vi "LiXiang's SRAM TESTING.vi"(8 "error in (no error)":errorcluster, 11 "DATA PATTERN":u8) -> (0 "错误输出":errorcluster, 3 "SEU number":u32)   [LabVIEW 2015]
doc: "演示连接TCP服务器、读取发送的数据并在图表上显示数据的方法。VI设计为TCP连接断开时停止。"
panel:
  out "布尔":bool
  out "SEU？":bool
  out "数组 2":i32[][](array[numeric])
  in  "行":u32
  out "数据输出":string
  in  "停止":bool
  # "地址"
  # "数据"
  # "0: 00\n1: 10\n2: 11"
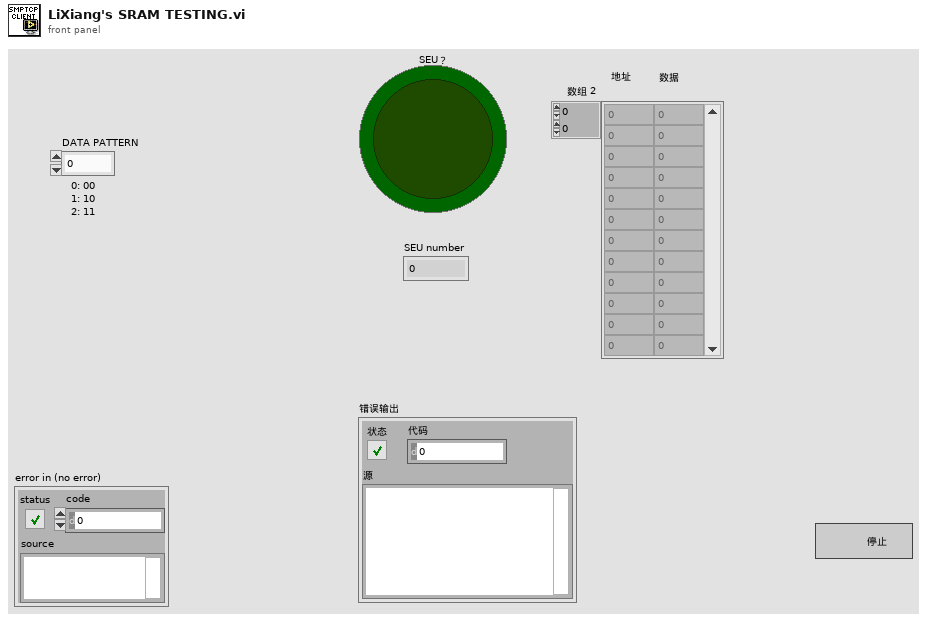
[diagram p1: front panel]
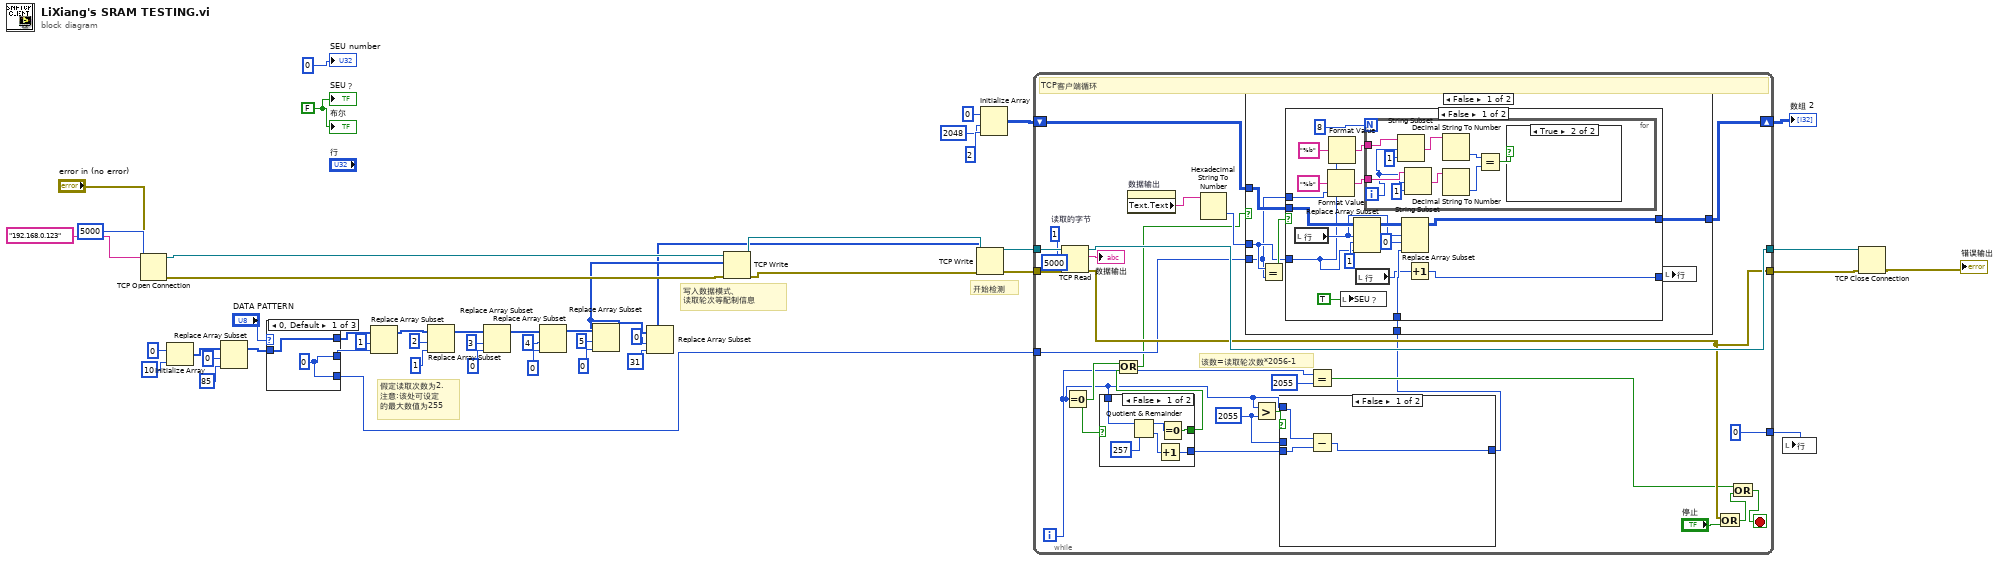
[diagram p0: block diagram]
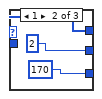
[diagram p2: hidden frame]
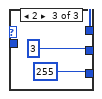
[diagram p3: hidden frame]
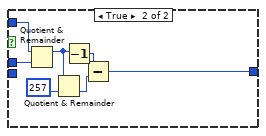
[diagram p4: hidden frame]
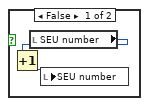
[diagram p5: hidden frame]
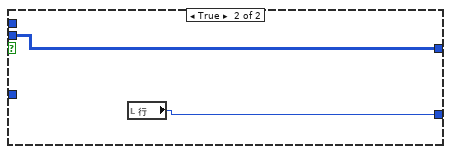
[diagram p6: hidden frame]
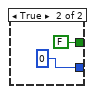
[diagram p8: hidden frame]
diagram:
  w7 = FALSE ("布尔")
  # "开始检测"
  # "写入数据模式、\n读取轮次等配制信息"
  # "假定读取次数为2.\n注意:该处可设定\n的最大数值为255"
  n1 = TCP Open Connection(address="192.168.0.123" ("地址"), remote port or service name=u16 5000 ("端口"), error in (no error)="error in (no error)") -> (connection ID=w25:refnum<k5>, error out=w24:errorcluster)  [unwired: 2 in]
  n2 = Initialize Array(u8 0 ("元素"), 10 ("维数大小")) -> (w43:u8[])
  n3 = Replace Array Subset(array=w43, new element=u8 85 ("新元素/子数组"), index=0 ("索引")) -> (w40:u8[])
  n4 = case shown="0, Default" "DATA PATTERN" {
    tunnel: w40 -> [w49 w52 w55]
    tunnel: [w49 w52 w55] -> w27
    tunnel: [w48 u8 2 ("新元素/子数组") u8 3 ("新元素/子数组")] -> w8
    tunnel: [w48 u32 170 ("新元素/子数组") u32 255 ("新元素/子数组")] -> w10
    frame 0, Default {
      w48 = u8 0 ("新元素/子数组")
    }
    frame 1 {
    }
    frame 2 {
    }
  }
  n5 = Replace Array Subset(array=w27, new element=w8, index=1 ("索引")) -> (w26:u8[])
  n6 = Replace Array Subset(array=w26, new element=u8 1 ("新元素/子数组"), index=2 ("索引")) -> (w36:u8[])
  n7 = Replace Array Subset(array=w36, new element=u8 0 ("新元素/子数组"), index=3 ("索引")) -> (w33:u8[])
  n8 = Replace Array Subset(array=w33, new element=u8 0 ("新元素/子数组"), index=4 ("索引")) -> (w30:u8[])
  n9 = Replace Array Subset(array=w30, new element=u8 0 ("新元素/子数组"), index=5 ("索引")) -> (w18:u8[])
  n10 = Replace Array Subset(array=w18, new element=u8 31 ("新元素/子数组"), index=0 ("索引")) -> (w17:u8[])
  n11 = TCP Write(connection ID=w25, data in=w18, error in (no error)=w24) -> (connection ID out=w23:refnum<k5>, error out=w5:errorcluster)  [unwired: 1 in, 1 out]
  n12 = TCP Write(connection ID=w23, data in=w17, error in (no error)=w5) -> (connection ID out=w21:refnum<k5>, error out=w22:errorcluster)  [unwired: 1 in, 1 out]
  n13 = Initialize Array(0 ("元素"), 2048 ("维数大小"), 2 ("维数大小")) -> (w12:i32[][])
  n14 = while {
    tunnel: w22 -> [w80]
    tunnel: w21 -> [w81]
    tunnel: [w77] -> w1
    tunnel: [w76] -> w3
    tunnel: w10 -> [w69]
    shift-right: [w62] -> w6
    shift-left: w12 -> [w65]
    tunnel: [u32 0 ("行")] -> w11
    i -> [w60]
    stop <- w73 stop-if-true
    w63 = 2055 ("y")
    w79 = 1  # 读取的字节
    # "该数=读取轮次数*2056-1"
    # "TCP客户端循环"
    n15 = TCP Read(connection ID=w81, bytes to read=w79, error in (no error)=w80, 9:5000 ("超时毫秒(25000)")) -> (connection ID out=w77:refnum<k5>, data out=→"数据输出":string, error out=w76:errorcluster)  [unwired: 1 in]
    n16 = Equal To 0?(x=w60) -> (x = 0?=w68:bool)
    n17 = case shown="False" w68 {
      tunnel: w60 -> [w131 _]
      tunnel: [w134 FALSE] -> w67
      tunnel: [w132 0] -> w58
      frame False {
        n18 = Quotient & Remainder(x=w131, y=257) -> (x-y*floor(x/y)=w135:i32, floor(x/y)=w133:i32)
        n19 = Increment(x=w133) -> (x+1=w132:i32)
        n20 = Equal To 0?(x=w135) -> (x = 0?=w134:bool)
      }
      frame True {
      }
    }
    n21 = Or(x=w68, y=w67) -> (x .or. y?=w66:bool)
    n22 = property on="数据输出" class="Str"() -> ("Text.Text"=w57:string)  [unwired: 2 in, 2 out]
    n23 = Hexadecimal String To Number(string=w57) -> (number=w70:u32)  [unwired: 2 in, 1 out]
    n24 = Greater?(x=w60, y=w63) -> (0:w64:bool)
    n25 = case shown="False" w64 {
      tunnel: w60 -> [w82 w91]
      tunnel: w63 -> [_ w90]
      tunnel: [w83 w86] -> w59
      tunnel: w58 -> [w84 _]
      frame False {
        n26 = Subtract(x=w82, y=w84) -> (x-y=w83:i32)
      }
      frame True {
        n27 = Quotient & Remainder(x=w91, y=w90) -> (x-y*floor(x/y)=w89:i32)  [unwired: 1 out]
        n28 = Quotient & Remainder(x=w89, y=257) -> (floor(x/y)=w87:i32)  [unwired: 1 out]
        n29 = Decrement(x=w89) -> (x-1=w85:i32)
        n30 = Subtract(x=w85, y=w87) -> (x-y=w86:i32)
      }
    }
    n31 = case shown="False" w66 {
      tunnel: w70 -> [w95 _]
      tunnel: w69 -> [w92 _]
      tunnel: w65 -> [w97 w130]
      tunnel: w59 -> [w96 _]
      tunnel: [w94 w130] -> w62
      frame False {
        n32 = Equal?(x=w95, y=w92) -> (x = y?=w98:bool)
        n33 = case shown="False" w98 {
          tunnel: w97 -> [w115 w129]
          tunnel: w96 -> [w110 _]
          tunnel: w95 -> [w103 _]
          tunnel: [w109 w129] -> w94
          tunnel: [w107 w128] -> w93
          tunnel: w92 -> [w100 _]
          frame False {
            n34 = local read "行"() -> (w112:u32)
            n35 = Format Value(format string="%b" ("格式字符串"), value (0)=w100) -> (output string=w99:string)  [unwired: 1 in]
            n36 = Format Value(format string="%b" ("格式字符串"), value (0)=w103) -> (output string=w102:string)  [unwired: 1 in]
            n37 = local write "SEU？"(TRUE ("SEU？")) -> ()
            n38 = Replace Array Subset(array=w115, new element=w103, index (row)=w112, index (col)=1 ("禁用的索引 (列)")) -> (w113:i32[][])
            n39 = local read "行"() -> (w108:u32)
            n40 = for {
              N: 8 -> [_]
              tunnel: w102 -> [w125]
              tunnel: w99 -> [w121]
              i -> [w120]
              n41 = String Subset(string=w125, offset (0)=w120, length (rest)=1 ("长度（剩余）")) -> (substring=w123:string)
              n42 = String Subset(string=w121, offset (0)=w120, length (rest)=1 ("长度（剩余）")) -> (substring=w119:string)
              n43 = Decimal String To Number(string=w123) -> (number=w118:i32)  [unwired: 2 in, 1 out]
              n44 = Decimal String To Number(string=w119) -> (number=w117:i32)  [unwired: 2 in, 1 out]
              n45 = Equal?(x=w118, y=w117) -> (x = y?=w116:bool)
              n46 = case shown="True" w116 {
                frame False {
                  n47 = local read "SEU number"() -> (w127:u32)
                  n48 = Increment(x=w127) -> (x+1=w126:u32)
                  n49 = local write "SEU number"(w126) -> ()
                }
                frame True {
                }
              }
            }
            n50 = Replace Array Subset(array=w113, new element=w110, index (row)=w112, index (col)=0 ("禁用的索引 (列)")) -> (w109:i32[][])
            n51 = Increment(x=w108) -> (x+1=w107:u32)
          }
          frame True {
            n52 = local read "行"() -> (w128:u32)
          }
        }
        n53 = local write "行"(w93) -> ()
      }
      frame True {
      }
    }
    n54 = Equal?(x=w60, y=2055) -> (x = y?=w75:bool)
    n55 = Or(x=w76, y="停止") -> (x .or. y?=w74:bool)
    n56 = Or(x=w75, y=w74) -> (x .or. y?=w73:bool)
  }
  "数组 2" <- w6
  n57 = local write "行"(w11) -> ()
  n58 = TCP Close Connection(connection ID=w1, error in (no error)=w3) -> (error out=→"错误输出":errorcluster)  [unwired: 1 in, 1 out]
  "SEU？" <- w7
  "SEU number" <- u32 0 ("SEU number")
  "布尔" <- w7
